vi "Start Session.vi"(8 "error in":errorcluster, 9 "Password":string, 10 "Username":string, 11 "Framework Engine in":refnum<class "Framework Engine.lvclass">) -> (0 "error out":errorcluster, 3 "Framework Engine out":refnum<class "Framework Engine.lvclass">)   [LabVIEW 2026, in "Framework Engine.lvclass"]
uses:
  Framework Engine.lvclass
  Framework Engine.lvclass/Framework Engine.ctl
  Services/Authentication Service/Authentication Service.lvclass
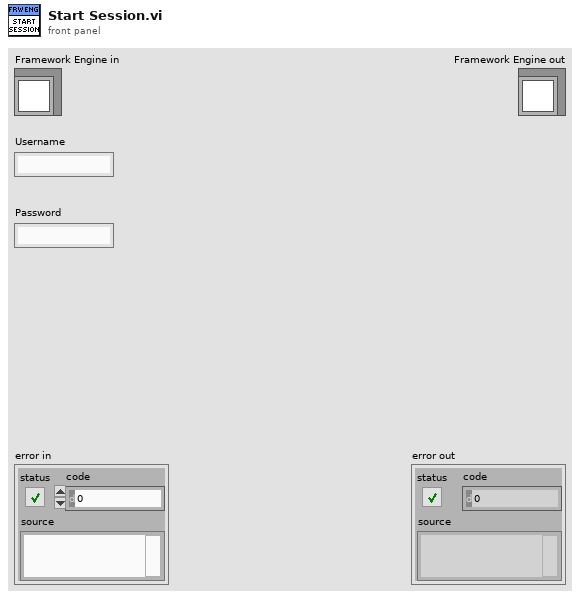
[diagram p1: front panel]
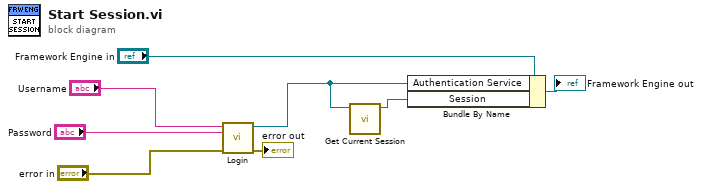
[diagram p0: block diagram]
diagram:
  n1 = call "Login.vi"("error in"="error in", "Password"="Password", "Username"="Username") -> ("error out"=→"error out":errorcluster, "Authentication Service"=w2:refnum<class "Authentication Service.lvclass">)  [unwired: 7 in]
  n2 = call "Get Current Session.vi"("Authentication Service"=w2) -> ("Current Session"=w1:refnum<class "Session.lvclass">)  [unwired: 10 in]
  n3 = Bundle By Name(cluster="Framework Engine in", "Authentication Service"=w2, "Session"=w1) -> (→"Framework Engine out":refnum<class "Framework Engine.lvclass">)
